vi "Read Command FIFO.vi"(8 "error in (no error)":errorcluster, 11 "Plugin in":refnum<class "Plugin.lvclass">) -> (0 "error out":errorcluster, 2 "Command FIFO Ref":T1, 3 "Plugin out":refnum<class "Plugin.lvclass">)   [LabVIEW 2016, in "Plugin.lvclass"]
uses:
  Plugin.lvclass
  Typdefs/Command FIFO Ref.ctl
  Typdefs/Plugin FIFO Data.ctl
  Typdefs/Plugin Commands.ctl
  <vilib>/NI Veristand/VeriStand Data/Byte Buffer/Byte Buffer.Pointers.ctl
  Plugin.lvclass/Plugin.ctl
  <vilib>/NI Veristand/VeriStand Data/Byte Buffer/Byte Buffer.lvclass
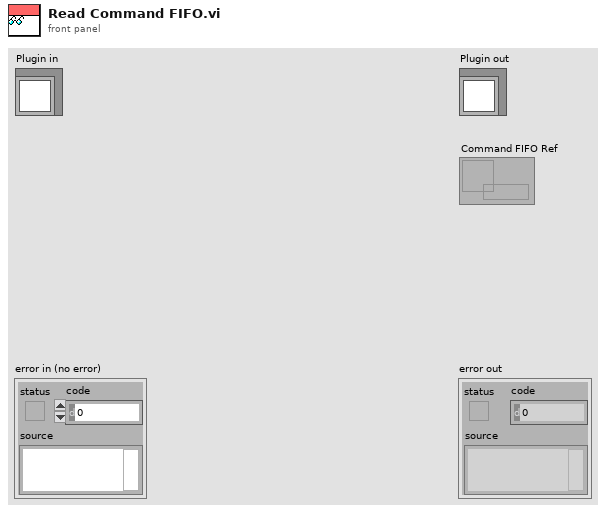
[diagram p1: front panel]
types:
  T1 = typedef "Command FIFO Ref.ctl" = refnum<k33>
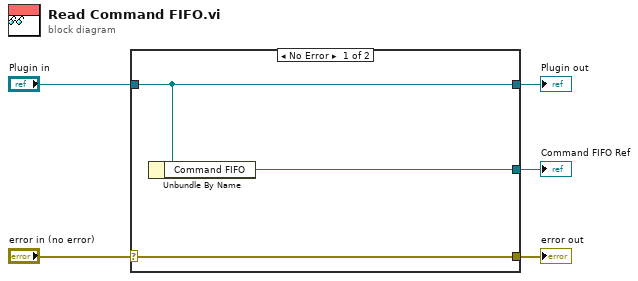
[diagram p0: block diagram]
diagram:
  n1 = case shown="No Error" "error in (no error)" {
    selector: "error in (no error)" -> [w8 w9]
    tunnel: [w8 w9] -> w4
    tunnel: [w7 w10] -> w2
    tunnel: "Plugin in" -> [w7 w10]
    tunnel: [w6 _] -> w1
    frame No Error {
      n2 = Unbundle By Name(w7) -> ("Command FIFO"=w6:T1)
    }
    frame Error {
    }
  }
  "error out" <- w4
  "Plugin out" <- w2
  "Command FIFO Ref" <- w1
